vi "saveDataNodeBegin.vi"(8 "error in (no error)":errorcluster, 9 "indent":i32, 10 "XML Refnum in":refnum<file>, 11 "FPGADMAChannelData in":refnum<class "FPGADMAChannelData.lvclass">) -> (0 "error out":errorcluster, 2 "XML Refnum out":refnum<file>, 3 "FPGADMAChannelData out":refnum<class "FPGADMAChannelData.lvclass">)   [LabVIEW 2013, in "FPGADMAChannelData.lvclass"]
doc: "Begins the process of saving a xceData Node to an XML formatted file."
uses:
  FPGADMAChannelData.lvclass
  FPGADMAChannelData.lvclass/FPGADMAChannelData.ctl
  xCE/xceNode/xceNode.lvclass
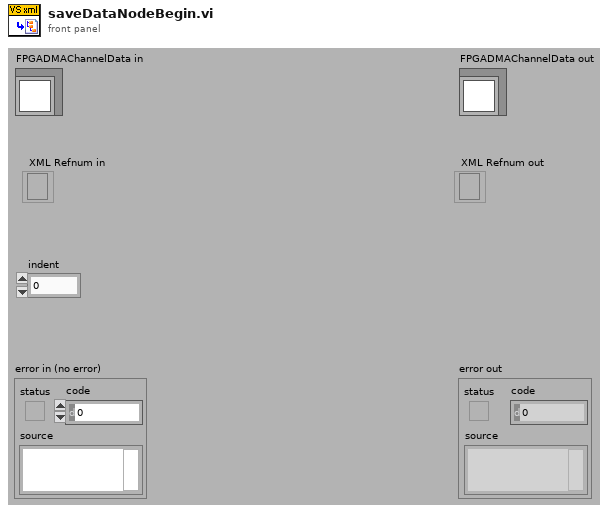
[diagram p1: front panel]
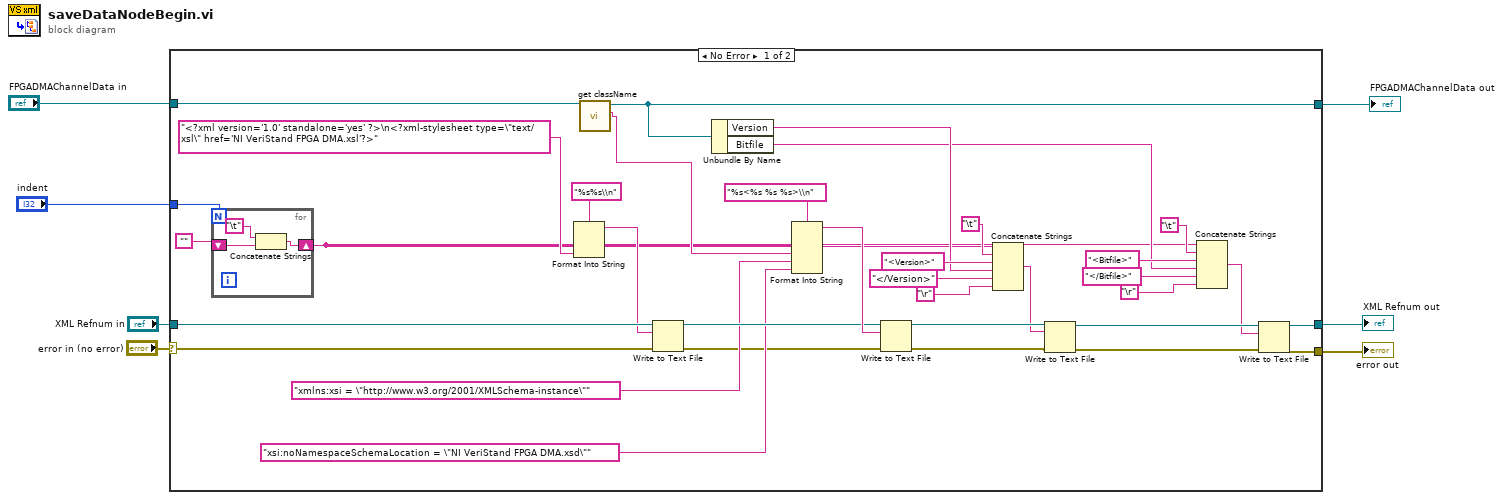
[diagram p0: block diagram]
diagram:
  n1 = case shown="No Error" "error in (no error)" {
    selector: "error in (no error)" -> [w34 w46]
    tunnel: "indent" -> [w41 _]
    tunnel: "XML Refnum in" -> [w36 w47]
    tunnel: "FPGADMAChannelData in" -> [w40 w48]
    tunnel: [w39 w48] -> w3
    tunnel: [w11 w47] -> w1
    tunnel: [w15 w46] -> w2
    frame No Error {
      n2 = for {
        N: w41 -> [_]
        shift-right: [w45] -> w8
        shift-left: "" -> [w44]
        n3 = Concatenate Strings("\t", w44) -> (w45:string)
      }
      n4 = Format Into String(format string="%s%s\\n", w8, "<?xml version='1.0' standalone='yes' ?>\n<?xml-stylesheet type=\"text/xsl\" href='NI VeriStand FPGA DMA.xsl'?>" ("format string")) -> (resulting string=w35:string)  [unwired: 2 in, 1 out]
      n5 = call "get className.vi"("xceNode in"=w40) -> ("Class name"=w9:string, "xceNode out"=w39:refnum<class "FPGADMAChannelData.lvclass">)  [unwired: 8 in, 1 out]
      n6 = Write to Text File(file (use dialog)=w36, text=w35, error in=w34) -> (refnum out=w31:refnum<file>, error out=w28:errorcluster)  [unwired: 1 in, 1 out]
      n7 = Unbundle By Name(w39) -> ("Version"=w23:string, "Bitfile"=w10:string)
      n8 = Format Into String(format string="%s<%s %s %s>\\n", w8, w9, "xmlns:xsi = \"http://www.w3.org/2001/XMLSchema-instance\"" ("format string"), "xsi:noNamespaceSchemaLocation = \"NI VeriStand FPGA DMA.xsd\"" ("format string")) -> (resulting string=w32:string)  [unwired: 2 in, 1 out]
      n9 = Write to Text File(file (use dialog)=w31, text=w32, error in=w28) -> (refnum out=w14:refnum<file>, error out=w12:errorcluster)  [unwired: 1 in, 1 out]
      n10 = Concatenate Strings(w8, "\t", "<Version>", w23, "</Version>" ("string"), "\r") -> (w13:string)
      n11 = Write to Text File(file (use dialog)=w14, text=w13, error in=w12) -> (refnum out=w21:refnum<file>, error out=w22:errorcluster)  [unwired: 1 in, 1 out]
      n12 = Concatenate Strings(w8, "\t", "<Bitfile>", w10, "</Bitfile>" ("string"), "\r") -> (w20:string)
      n13 = Write to Text File(file (use dialog)=w21, text=w20, error in=w22) -> (refnum out=w11:refnum<file>, error out=w15:errorcluster)  [unwired: 1 in, 1 out]
    }
    frame Error {
    }
  }
  "error out" <- w2
  "FPGADMAChannelData out" <- w3
  "XML Refnum out" <- w1
